vi "Convert Digital to Analog Waveform Multi Channel.vi"(6 "Channels index":i32[](array[numeric]), 8 "full scale range":dbl=10.0 format="%#_13g", 9 "Number of samples":u32, 10 "Sample rate":dbl, 11 "Digital Waveform":u32[](array[numeric])) -> (3 "Waveforms":waveform(dbl)[](array[waveform]))   [LabVIEW 2021]
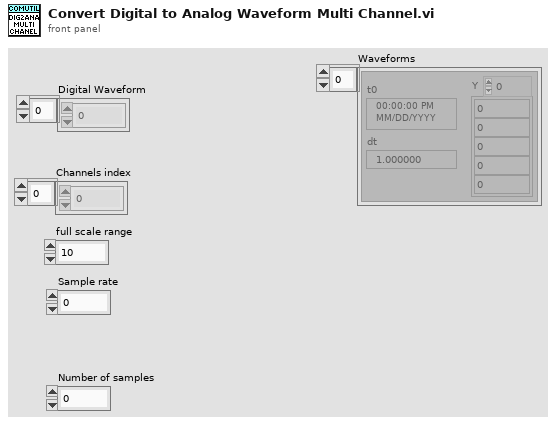
[diagram p1: front panel]
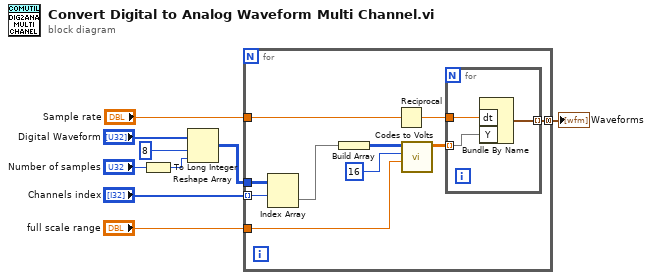
[diagram p0: block diagram]
diagram:
  n1 = To Long Integer(number="Number of samples") -> (32bit integer=w1:i32)
  n2 = Reshape Array("Digital Waveform", 8 ("dimension size"), w1) -> (w7:u32[][])
  n3 = for {
    tunnel: "Sample rate" -> [w19]
    tunnel: [w15] -> w5 mode=concatenating
    tunnel: w7 -> [w14]
    tunnel: "Channels index" -> [w12] mode=indexing
    tunnel: "full scale range" -> [w10]
    n4 = Index Array(array=w14, index (row)=w12) -> (element=w13:u32[])  [unwired: 1 in]
    n5 = Build Array(w13) -> (w11:u32[][])
    n6 = Reciprocal(x=w19) -> (1/x=w18:dbl)
    n7 = call "Codes to Volts.vi"("full scale range"=w10, "number of bits"=16, "data"=w11) -> ("scaled data"=w16:dbl[][])  [unwired: 7 in, 1 out]
    n8 = for {
      tunnel: w18 -> [w22]
      tunnel: w16 -> [w21] mode=indexing
      tunnel: [w20] -> w15 mode=indexing
      n9 = Bundle By Name("dt"=w22, "Y"=w21) -> (w20:waveform(dbl))  [unwired: 1 in]
    }
  }
  "Waveforms" <- w5
